vi "Scan Hydra - Test.vi"(2 "error in":errorcluster) -> (0 "error out":errorcluster, 1 "next scan":dbl[](array[numeric]) format="%.2f")   [LabVIEW 2019]
uses:
  Global Variables/Global_Variables.vi
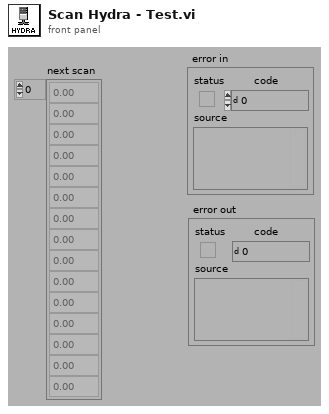
[diagram p1: front panel]
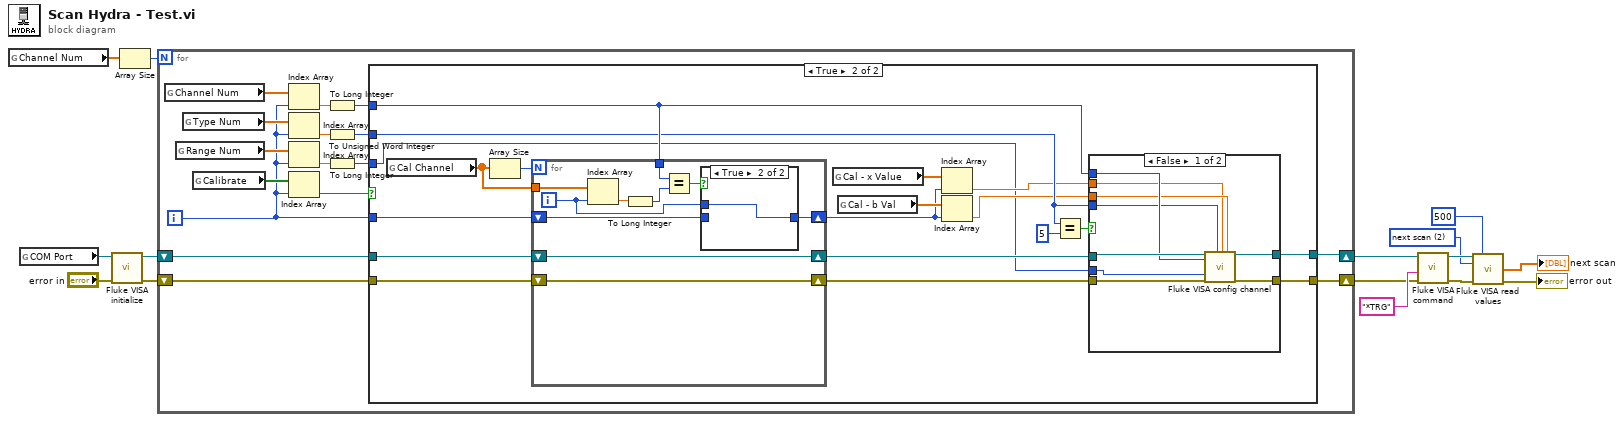
[diagram p0: block diagram]
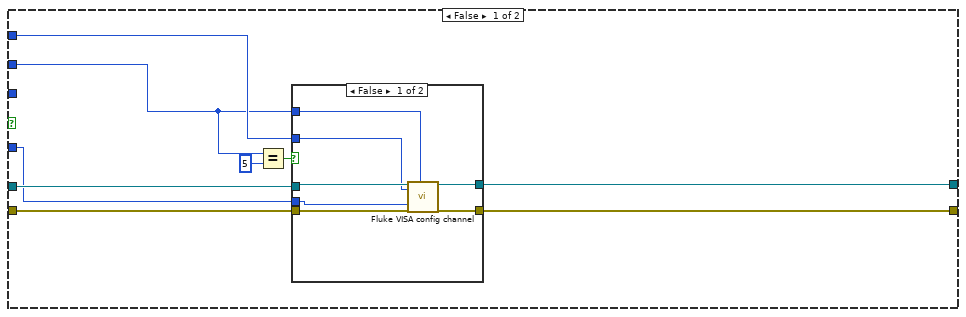
[diagram p2: hidden frame]
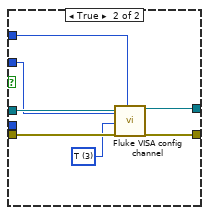
[diagram p3: hidden frame]
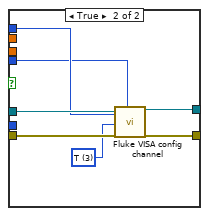
[diagram p5: hidden frame]
diagram:
  w10 = 2 items=["min, max, & last", "monitor value", "next scan", "current total"] ("values to read")
  n1 = global read "Global_Variables.vi" "Channel Num"() -> (w6:dbl[])
  n2 = global read "Global_Variables.vi" "COM Port"() -> (w7:refnum<visa-resource-name>)
  n3 = call "Fluke VISA initialize.vi"("error in (no error)"="error in", "Hydra VISA in"=w7) -> ("error out"=w3:errorcluster, "Hydra VISA out"=w4:refnum<visa-resource-name>)  [unwired: 3 in, 1 out]
  n4 = Array Size(array=w6) -> (size(s)=w5:i32)
  n5 = for {
    N: w5 -> [_]
    shift-right: [w21] -> w1
    shift-left: w4 -> [w23]
    shift-right: [w20] -> w2
    shift-left: w3 -> [w22]
    i -> [w16]
    n6 = global read "Global_Variables.vi" "Channel Num"() -> (w31:dbl[])
    n7 = global read "Global_Variables.vi" "Range Num"() -> (w29:dbl[])
    n8 = global read "Global_Variables.vi" "Type Num"() -> (w30:dbl[])
    n9 = global read "Global_Variables.vi" "Calibrate"() -> (w25:bool[])
    n10 = Index Array(array=w31, index=w16) -> (element=w28:dbl)
    n11 = Index Array(array=w30, index=w16) -> (element=w27:dbl)
    n12 = Index Array(array=w29, index=w16) -> (element=w26:dbl)
    n13 = Index Array(array=w25, index=w16) -> (element=w24:bool)
    n14 = To Long Integer(number=w28) -> (32bit integer=w17:i32)
    n15 = To Unsigned Word Integer(number=w27) -> (unsigned 16bit integer=w18:u16)
    n16 = To Long Integer(number=w26) -> (32bit integer=w19:i32)
    n17 = case shown="True" w24 {
      tunnel: w23 -> [w37 w66]
      tunnel: w22 -> [w38 w65]
      tunnel: [w36 w70] -> w21
      tunnel: [w35 w71] -> w20
      tunnel: w19 -> [_ w55]
      tunnel: w18 -> [w33 w58]
      tunnel: w17 -> [w34 w59]
      tunnel: w16 -> [w32 w68]
      frame False {
        n18 = Equal?(x=w33, y=u16 5) -> (x = y?=w40:bool)
        n19 = case shown="False" w40 {
          tunnel: w37 -> [w46 w53]
          tunnel: w38 -> [w47 w54]
          tunnel: [w44 w52] -> w36
          tunnel: [w45 w51] -> w35
          tunnel: w34 -> [w43 w49]
          tunnel: w33 -> [w42 w48]
          tunnel: w32 -> [w41 _]
          frame False {
            n20 = call "Fluke VISA config channel.vi"("Hydra VISA in"=w46, "channel"=w43, "range (auto:0)"=w41, "error in (no error)"=w47, "function (off:0)"=w42) -> ("Hydra VISA out"=w44:refnum<visa-resource-name>, "error out"=w45:errorcluster)  [unwired: 13 in]
          }
          frame True {
            w50 = 3 items=["J", "K", "E", "T", "N", "R", "S", "B", "C"] ("thermocouple (J:0)")
            n21 = call "Fluke VISA config channel.vi"("Hydra VISA in"=w53, "channel"=w49, "thermocouple (J:0)"=w50, "error in (no error)"=w54, "function (off:0)"=w48) -> ("Hydra VISA out"=w52:refnum<visa-resource-name>, "error out"=w51:errorcluster)  [unwired: 13 in]
          }
        }
      }
      frame True {
        n22 = global read "Global_Variables.vi" "Cal Channel"() -> (w67:dbl[])
        n23 = Array Size(array=w67) -> (size(s)=w69:i32)
        n24 = for {
          N: w69 -> [_]
          shift-right: [w75] -> w62
          shift-left: w68 -> [w76]
          tunnel: w67 -> [w83]
          tunnel: w59 -> [w82]
          shift-right: [w79] -> w61
          shift-left: w66 -> [w79]
          shift-right: [w78] -> w60
          shift-left: w65 -> [w78]
          i -> [w74]
          n25 = Index Array(array=w83, index=w74) -> (element=w81:dbl)
          n26 = To Long Integer(number=w81) -> (32bit integer=w80:i32)
          n27 = Equal?(x=w82, y=w80) -> (x = y?=w77:bool)
          n28 = case shown="True" w77 {
            tunnel: w76 -> [w84 _]
            tunnel: [w84 w85] -> w75
            tunnel: w74 -> [_ w85]
            frame False {
            }
            frame True {
            }
          }
        }
        n29 = global read "Global_Variables.vi" "Cal - x Value"() -> (w64:dbl[])
        n30 = global read "Global_Variables.vi" "Cal - b Val"() -> (w63:dbl[])
        n31 = Index Array(array=w64, index=w62) -> (element=w57:dbl)
        n32 = Index Array(array=w63, index=w62) -> (element=w56:dbl)
        n33 = Equal?(x=w58, y=u16 5) -> (x = y?=w73:bool)
        n34 = case shown="False" w73 {
          tunnel: w61 -> [w93 w100]
          tunnel: w60 -> [w94 w101]
          tunnel: [w91 w99] -> w70
          tunnel: [w92 w98] -> w71
          tunnel: w59 -> [w90 w96]
          tunnel: w58 -> [w89 w95]
          tunnel: w57 -> [w87 _]
          tunnel: w56 -> [w88 _]
          tunnel: w55 -> [w86 _]
          frame False {
            n35 = call "Fluke VISA config channel.vi"("Hydra VISA in"=w93, "channel"=w90, "range (auto:0)"=w86, "error in (no error)"=w94, "function (off:0)"=w89, "Mx scaling"=w87, "+ B scaling"=w88) -> ("Hydra VISA out"=w91:refnum<visa-resource-name>, "error out"=w92:errorcluster)  [unwired: 11 in]
          }
          frame True {
            w97 = 3 items=["J", "K", "E", "T", "N", "R", "S", "B", "C"] ("thermocouple (J:0)")
            n36 = call "Fluke VISA config channel.vi"("Hydra VISA in"=w100, "channel"=w96, "thermocouple (J:0)"=w97, "error in (no error)"=w101, "function (off:0)"=w95) -> ("Hydra VISA out"=w99:refnum<visa-resource-name>, "error out"=w98:errorcluster)  [unwired: 13 in]
          }
        }
      }
    }
  }
  n37 = call "Fluke VISA command.vi"("error in (no error)"=w2, "Single Command"="*TRG", "Hydra VISA in"=w1) -> ("error out"=w13:errorcluster, "Hydra VISA out"=w14:refnum<visa-resource-name>)  [unwired: 3 in, 2 out]
  n38 = call "Fluke VISA read values.vi"("Hydra VISA in"=w14, "Byte Count"=u32 500, "values to read"=w10, "error in (no error)"=w13) -> ("next scan"=→"next scan":dbl[], "error out"=→"error out":errorcluster)  [unwired: 4 in, 6 out]
